vi "BuildTableForSignals.vi"() -> ()   [LabVIEW 2019]
panel:
  in  "stop":bool
  out "Mean":dbl
  out "Waveform Graph":dynamicdata(graph)
  in  "Simulate or not":bool
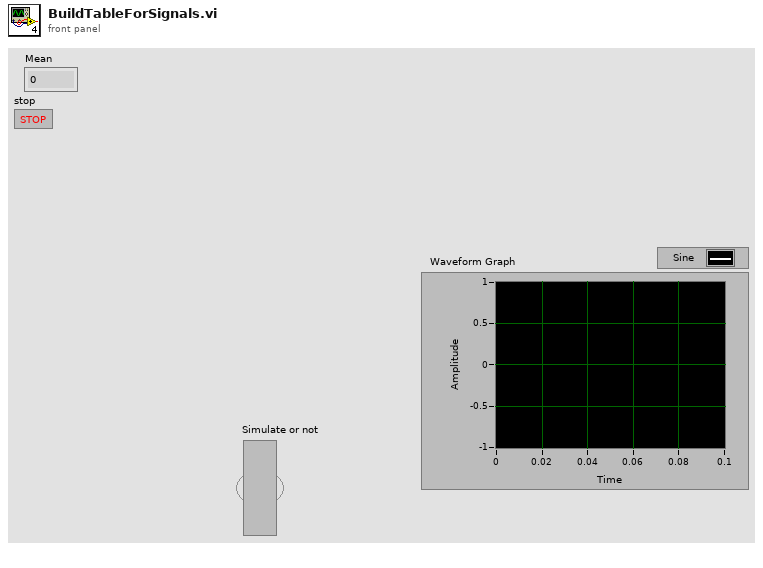
[diagram p1: front panel]
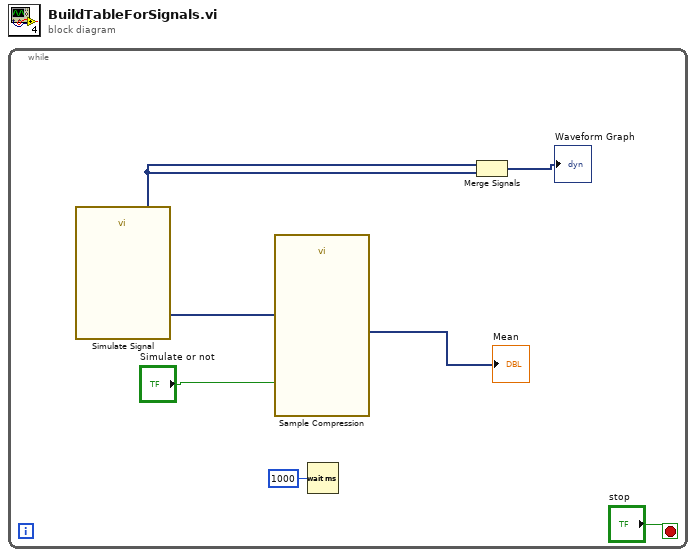
[diagram p0: block diagram]
diagram:
  n1 = while {
    stop <- "stop" stop-if-true
    n2 = call "Simulate Signal"() -> ("Sine"=w3:dynamicdata)  [unwired: 14 in, 1 out]
    n3 = call "Sample Compression"("Enable"="Simulate or not", "Signals"=w3) -> ("Mean"=→"Mean":dynamicdata)  [unwired: 7 in, 2 out]
    n4 = Wait (ms)(milliseconds to wait=u32 1000) -> ()  [unwired: 1 out]
    n5 = Merge Signals(w3, w3) -> (→"Waveform Graph":dynamicdata)
  }
